vi "PKG_IMC_Open.vi"(10 "imcid":i32, 11 "netcardsel":i32) -> (3 "function return":u32)   [LabVIEW 2018, in "IMC_Pkg4xxx.lvlib"]
doc: "PKG_IMC_Open (int netcardsel, int imcid) ;"
uses:
  IMC_Pkg4xxx.lvlib
  IMC_Pkg4xxx.dll
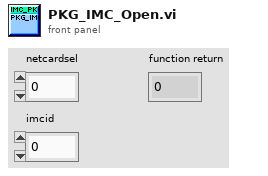
[diagram p1: front panel]
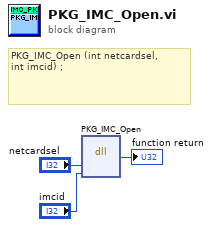
[diagram p0: block diagram]
diagram:
  # "PKG_IMC_Open (int netcardsel,\t\t\t\t\t\t\t\t\tint imcid) ;"
  n1 = dll-call lib="PTH2\\abs D做的项目航天测量驱动电机IMCAppincLabview32\nIMC_Pkg4xxx.*" fn="PKG_IMC_Open"("netcardsel"="netcardsel", "imcid"="imcid") -> (→"function return":u32)  [unwired: 5 in, 2 out]
